vi "Test FIFO Config flatten.vi"() -> ()   [LabVIEW 2021]
uses:
  typedef/FIFO Config.ctl
  <vilib>/CIF Foundation/CIF Utilities/DataTypes/Flatten U64.vi
  <vilib>/CIF Foundation/CIF Utilities/DataTypes/Unflatten U64.vi
  <userlib>/_OpenG.lib/numeric/numeric.llb/Random Number Within Range - DBL__ogtk.vi
  <userlib>/_OpenG.lib/numeric/numeric.llb/openg_numeric__ogtk.lvlib
  ChannelCommon.lvlib
panel:
  out "FIFO Config out":T1
  out "Pass":bool
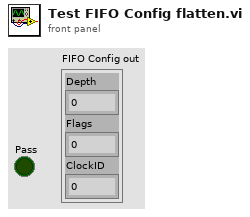
[diagram p1: front panel]
types:
  T1 = typedef "ChannelCommon.lvlib/FIFO Config.ctl" = cluster{"Depth":u64, "Flags":u64, "ClockID":u8}
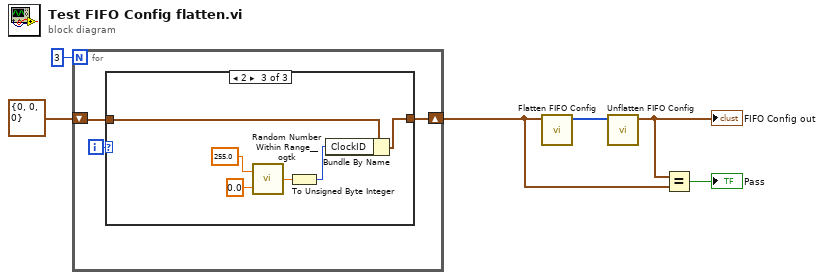
[diagram p0: block diagram]
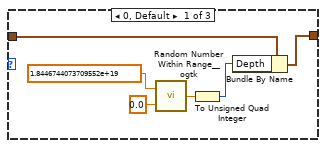
[diagram p2: hidden frame]
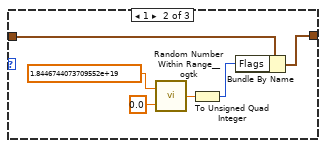
[diagram p3: hidden frame]
diagram:
  n1 = for {
    N: 3 -> [_]
    shift-right: [w7] -> w2
    shift-left: T1 {"Depth"=0, "Flags"=0, "ClockID"=0} ("FIFO Config in") -> [w8]
    i -> [w9]
    n2 = case shown="2" w9 {
      tunnel: w8 -> [w15 w21 w27]
      tunnel: [w10 w16 w22] -> w7
      frame 0, Default {
        n3 = call-poly <userlib>:"Random Number Within Range__ogtk.vi"("High"=1.8446744073709552e+19, "Low"=0.0) -> ("Random Number"=w12:dbl)  [unwired: 3 in]
        n4 = To Unsigned Quad Integer(1:w12) -> (0:w11:u64)
        n5 = Bundle By Name(cluster=w15, "Depth"=w11) -> (w10:T1)
      }
      frame 1 {
        n6 = call-poly <userlib>:"Random Number Within Range__ogtk.vi"("High"=1.8446744073709552e+19, "Low"=0.0) -> ("Random Number"=w18:dbl)  [unwired: 3 in]
        n7 = To Unsigned Quad Integer(1:w18) -> (0:w17:u64)
        n8 = Bundle By Name(cluster=w21, "Flags"=w17) -> (w16:T1)
      }
      frame 2 {
        n9 = call-poly <userlib>:"Random Number Within Range__ogtk.vi"("High"=255.0, "Low"=0.0) -> ("Random Number"=w24:dbl)  [unwired: 3 in]
        n10 = To Unsigned Byte Integer(number=w24) -> (unsigned 8bit integer=w23:u8)
        n11 = Bundle By Name(cluster=w27, "ClockID"=w23) -> (w22:T1)
      }
    }
  }
  n12 = call "Flatten FIFO Config.vi"("FIFO Config in"=w2) -> ("Flattened Data out"=w1:u8[])  [unwired: 10 in]
  n13 = call "Unflatten FIFO Config.vi"("Flattened Data in"=w1) -> ("FIFO Config out"=w3:T1)  [unwired: 9 in, 1 out]
  "FIFO Config out" <- w3
  n14 = Equal?(x=w3, y=w2) -> (x = y?=→"Pass":bool)
